vi "OpenIVIsamplePowersupply.vi"(2 "logical name (\"SamplePowerSupply\")":string="SamplePowerSupply", 3 "channel name (\"CHANNEL1\")":string="CHANNEL1") -> (0 "error in (no error)":errorcluster, 1 "instrument handle":refnum<k15>)   [LabVIEW 2010]
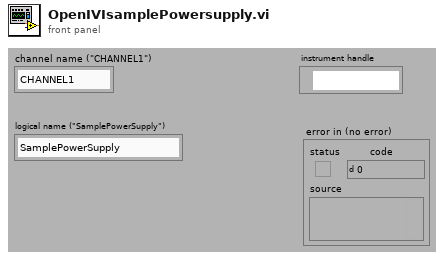
[diagram p1: front panel]
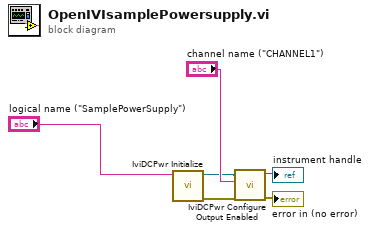
[diagram p0: block diagram]
diagram:
  n1 = call <vilib>:"IviDCPwr Initialize.vi"("logical name (\"SamplePowerSupply\")"="logical name (\"SamplePowerSupply\")") -> ("error out"=w1:errorcluster, "instrument handle"=w2:refnum<k15>)  [unwired: 3 in, 6 out]
  n2 = call <vilib>:"IviDCPwr Configure Output Enabled.vi"("error in (no error)"=w1, "channel name (\"CHANNEL1\")"="channel name (\"CHANNEL1\")", "instrument handle"=w2) -> ("error out"=→"error in (no error)":errorcluster, "instrument handle out"=→"instrument handle":refnum<k15>)  [unwired: 1 in, 6 out]
